vi "ble_rsp_attclient_read_by_handle.vi"(7 "Read long?(T)":bool=TRUE, 8 "error in (no error)":errorcluster, 11 "COM Bluegiga in":refnum<visa-resource-name>) -> (0 "error out":errorcluster, 1 "success?":bool, 2 "full message package":u8[](array[numeric]), 3 "COM Bluegiga out":refnum<visa-resource-name>)   [LabVIEW 2013]
uses:
  type_def/message_class.ctl
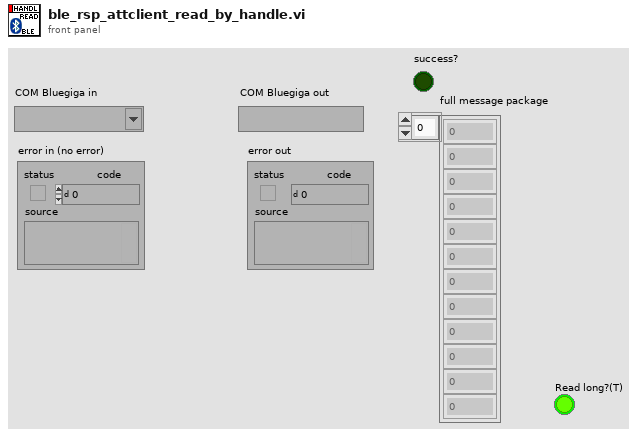
[diagram p1: front panel]
types:
  T1 = typedef "message_class.ctl" = u8
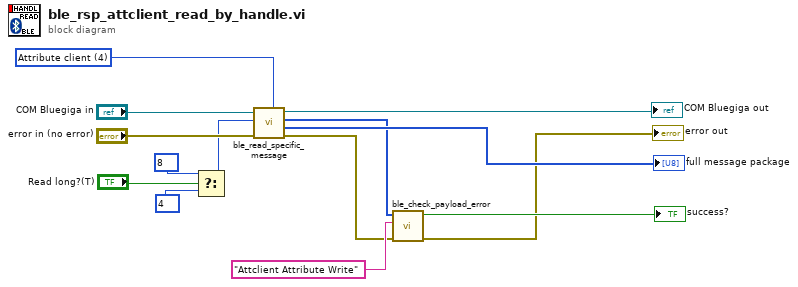
[diagram p0: block diagram]
diagram:
  w14 = T1 4 items=["System", "Persistent Store", "Attribute database", "Connection", "Attribute client", "Security Manager", "Generic Access Profile", "Hardware"] ("Command Class (System)")
  n1 = Select(t=u8 8 ("Message ID (0x00)"), s="Read long?(T)", f=u8 4 ("Message ID (0x00)")) -> (s? t:f=w2:u8)
  n2 = call "ble_read_specific_message.vi"("Command Class (System)"=w14, "error in (no error)"="error in (no error)", "Message ID (0x00)"=w2, "COM Bluegiga in"="COM Bluegiga in") -> ("error out"=w7:errorcluster, "full message package"=→"full message package":u8[], "specific payload"=w8:u8[], "COM Bluegiga out"=→"COM Bluegiga out":refnum<visa-resource-name>)  [unwired: 3 in, 1 out]
  n3 = call "ble_check_payload_error.vi"("error in (no error)"=w7, "error source"="Attclient Attribute Write", "payload"=w8) -> ("error out"=→"error out":errorcluster, "success?"=→"success?":bool)  [unwired: 7 in]
